vi "gfitsio-write-history.vi"(8 "error in (no error)":errorcluster, 9 "history":string, 11 "gfits refnum":T1) -> (0 "error out":errorcluster, 3 "dup gfits refnum":T1)   [LabVIEW 2019, in "gfitsio.lvlib"]
doc: "Append a HISTORY keyword to the current HDU. The comment string will be continued over multiple keywords if it is longer than 70 characters."
uses:
  gfitsio.lvlib
  gfitsio-refnum.ctl
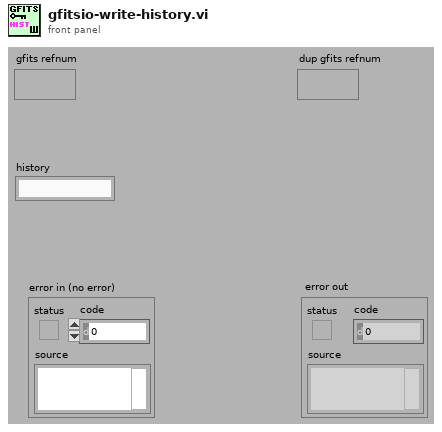
[diagram p1: front panel]
types:
  T1 = typedef "gfitsio.lvlib/gfitsio-refnum.ctl" = refnum<k1>
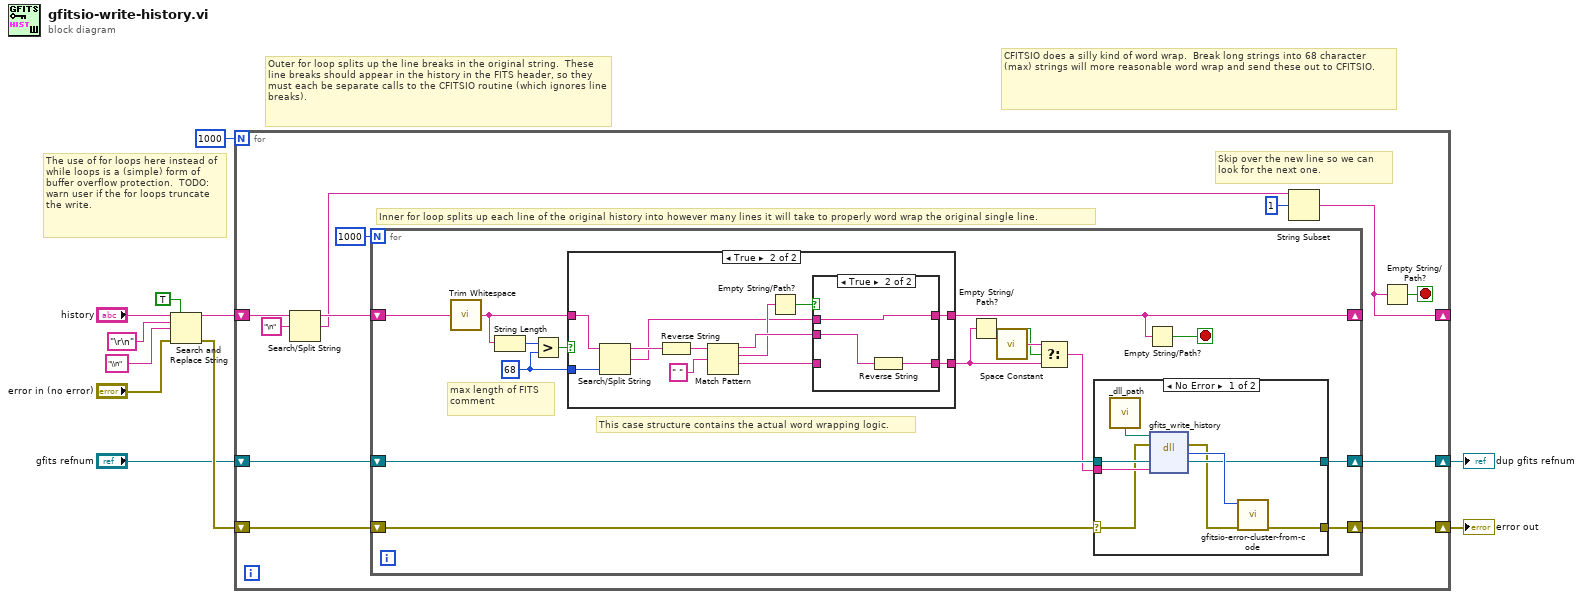
[diagram p0: block diagram]
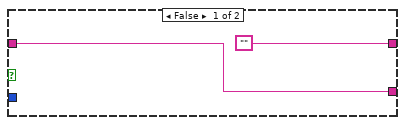
[diagram p3: hidden frame]
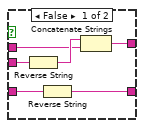
[diagram p4: hidden frame]
diagram:
  # "The use of for loops here instead of while loops is a (simple) form of buffer overflow protection.  TODO:  warn user if the for loops truncate the write."
  # "Outer for loop splits up the line breaks in the original string.  These line breaks should appear in the history in the FITS header, so they must each be separate calls to the CFITSIO routine (which ignores line breaks)."
  # "CFITSIO does a silly kind of word wrap.  Break long strings into 68 character (max) strings will more reasonable word wrap and send these out to CFITSIO."
  n1 = Search and Replace String(replace all?=TRUE ("replace all? (F)"), input string="history", search string="\r\n", replace string="\\n" ("replace string (\"\")"), error in="error in (no error)") -> (result string=w8:string, error out=w7:errorcluster)  [unwired: 3 in, 2 out]
  n2 = for {
    N: 1000 -> [_]
    shift-right: [w18] -> _
    shift-left: w8 -> [w23]
    shift-right: [w17] -> w3
    shift-left: "gfits refnum" -> [w16]
    shift-right: [w15] -> w4
    shift-left: w7 -> [w14]
    stop <- w13 stop-if-true
    # "Inner for loop splits up each line of the original history into however many lines it will take to properly word wrap the original single line."
    # "Skip over the new line so we can look for the next one."
    n3 = Search/Split String(string=w23, search string/char (-)="\n" ("regular expression")) -> (substring before match=w21:string, match + rest of string=w19:string)  [unwired: 1 in, 1 out]
    n4 = for {
      N: 1000 -> [_]
      shift-right: [w38] -> _
      shift-left: w21 -> [w31]
      shift-right: [w27] -> w17
      shift-left: w16 -> [w26]
      shift-right: [w28] -> w15
      shift-left: w14 -> [w29]
      stop <- w24 stop-if-true
      w36 = 68 ("length (rest)")
      # "This case structure contains the actual word wrapping logic."
      # "max length of FITS comment"
      n5 = call <vilib>:"Trim Whitespace.vi"("string"=w31) -> ("trimmed string"=w30:string)  [unwired: 1 in]
      n6 = String Length(string=w30) -> (length=w37:i32)
      n7 = Greater?(x=w37, y=w36) -> (0:w35:bool)
      n8 = case shown="True" w35 {
        tunnel: ["" w57] -> w38
        tunnel: [w50 w53] -> w32
        tunnel: w30 -> [w50 w52]
        tunnel: w36 -> [_ w51]
        frame False {
        }
        frame True {
          n9 = Search/Split String(string=w52, offset (0)=w51) -> (substring before match=w59:string, match + rest of string=w56:string)  [unwired: 1 in, 1 out]
          n10 = Reverse String(1:w59) -> (0:w62:string)
          n11 = Match Pattern(string=w62, regular expression=" ") -> (before substring=w60:string, match substring=w58:string, after substring=w54:string)  [unwired: 1 in, 1 out]
          n12 = Empty String/Path?(string/path=w58) -> (empty?=w55:bool)
          n13 = case shown="True" w55 {
            tunnel: w60 -> [w68 w69]
            tunnel: [w66 w71] -> w57
            tunnel: w56 -> [w65 w71]
            tunnel: w54 -> [w64 _]
            tunnel: [w63 w70] -> w53
            frame False {
              n14 = Reverse String(1:w68) -> (0:w67:string)
              n15 = Reverse String(1:w64) -> (0:w63:string)
              n16 = Concatenate Strings(w67, w65) -> (w66:string)
            }
            frame True {
              n17 = Reverse String(1:w69) -> (0:w70:string)
            }
          }
        }
      }
      n18 = Empty String/Path?(string/path=w32) -> (empty?=w33:bool)
      n19 = call <vilib>:"Space Constant.vi"() -> ("String"=w34:string)
      n20 = Select(t=w34, s=w33, f=w32) -> (s? t:f=w25:string)
      n21 = case shown="No Error" w29 {
        selector: w29 -> [w41 w48]
        tunnel: [w45 w48] -> w28
        tunnel: w26 -> [w42 w47]
        tunnel: [w43 w47] -> w27
        tunnel: w25 -> [w44 _]
        frame No Error {
          n22 = call "_dll_path.vi"() -> ("Path"=w39:path)  [unwired: 1 in]
          n23 = dll-call lib="?" fn="gfits_write_history"(path in=w39, error in=w41, "refnum"=w42, "comment"=w44) -> (error out=w40:errorcluster, "return type"=w46:i32, "refnum"=w43:T1)  [unwired: 2 in, 1 out]
          n24 = call "gfitsio-error-cluster-from-code.vi"("error in (no error)"=w40, "error code"=w46) -> ("error out"=w45:errorcluster)  [unwired: 9 out]
        }
        frame Error {
        }
      }
      n25 = Empty String/Path?(string/path=w38) -> (empty?=w24:bool)
    }
    n26 = String Subset(string=w19, offset (0)=1) -> (substring=w18:string)  [unwired: 1 in]
    n27 = Empty String/Path?(string/path=w18) -> (empty?=w13:bool)
  }
  "error out" <- w4
  "dup gfits refnum" <- w3
